vi "Scanner Box Setup.vi"(8 "error in":errorcluster, 11 "VISA resource name":refnum<visa-resource-name>) -> (0 "error out":errorcluster, 3 "VISA resource name out":refnum<visa-resource-name>)   [LabVIEW 2011, in "GPT-9000.lvlib"]
uses:
  <instrlib>/GPT-9000/GPT-9000.lvlib
panel:
  out "Error Message":string
  out "ID Return String":string
  in  "Clear Error(True)":bool=TRUE
  in  "ID Query (True)":bool=TRUE
  in  "Configure RS232 Baud Rate":u32(ring)=115200 items=["9600"=9600, "19200"=19200, "38400"=38400, "57600"=57600, "115200"=115200]
  out "Return the Lo Set Value":u32 format="%08x"
  out "Return the Hi Set Value":u32 format="%08x"
  in  "Number for MANU":i32=1 min=1 max=100 step=1
  in  "CH8_4":enum32{"HI", "LO", "OFF"}(radio)=enum."OFF" caption="CH8"
  in  "CH7_4":enum32{"HI", "LO", "OFF"}(radio)=enum."OFF" caption="CH7"
  in  "CH6_4":enum32{"HI", "LO", "OFF"}(radio)=enum."OFF" caption="CH6"
  in  "CH5_4":enum32{"HI", "LO", "OFF"}(radio)=enum."OFF" caption="CH5"
  in  "CH4_4":enum32{"HI", "LO", "OFF"}(radio)=enum."OFF" caption="CH4"
  in  "CH3_4":enum32{"HI", "LO", "OFF"}(radio)=enum."OFF" caption="CH3"
  in  "CH2_4":enum32{"HI", "LO", "OFF"}(radio)=enum."OFF" caption="CH2"
  in  "CH1_4":enum32{"HI", "LO", "OFF"}(radio)=enum."OFF" caption="CH1"
  in  "CH8_3":enum32{"HI", "LO", "OFF"}(radio)=enum."OFF" caption="CH8"
  in  "CH7_3":enum32{"HI", "LO", "OFF"}(radio)=enum."OFF" caption="CH7"
  in  "CH6_3":enum32{"HI", "LO", "OFF"}(radio)=enum."OFF" caption="CH6"
  in  "CH5_3":enum32{"HI", "LO", "OFF"}(radio)=enum."OFF" caption="CH5"
  in  "CH4_3":enum32{"HI", "LO", "OFF"}(radio)=enum."OFF" caption="CH4"
  in  "CH3_3":enum32{"HI", "LO", "OFF"}(radio)=enum."OFF" caption="CH3"
  in  "CH2_3":enum32{"HI", "LO", "OFF"}(radio)=enum."OFF" caption="CH2"
  in  "CH1_3":enum32{"HI", "LO", "OFF"}(radio)=enum."OFF" caption="CH1"
  in  "CH8_2":enum32{"HI", "LO", "OFF"}(radio)=enum."OFF" caption="CH8"
  in  "CH7_2":enum32{"HI", "LO", "OFF"}(radio)=enum."OFF" caption="CH7"
  in  "CH6_2":enum32{"HI", "LO", "OFF"}(radio)=enum."OFF" caption="CH6"
  in  "CH5_2":enum32{"HI", "LO", "OFF"}(radio)=enum."OFF" caption="CH5"
  in  "CH4_2":enum32{"HI", "LO", "OFF"}(radio)=enum."OFF" caption="CH4"
  in  "CH3_2":enum32{"HI", "LO", "OFF"}(radio)=enum."OFF" caption="CH3"
  in  "CH2_2":enum32{"HI", "LO", "OFF"}(radio)=enum."OFF" caption="CH2"
  in  "CH1_2":enum32{"HI", "LO", "OFF"}(radio)=enum."OFF" caption="CH1"
  in  "CH8_1":enum32{"HI", "LO", "OFF"}(radio)=enum."OFF" caption="CH8"
  in  "CH7_1":enum32{"HI", "LO", "OFF"}(radio)=enum."OFF" caption="CH7"
  in  "CH6_1":enum32{"HI", "LO", "OFF"}(radio)=enum."OFF" caption="CH6"
  in  "CH5_1":enum32{"HI", "LO", "OFF"}(radio)=enum."OFF" caption="CH5"
  in  "CH4_1":enum32{"HI", "LO", "OFF"}(radio)=enum."OFF" caption="CH4"
  in  "CH3_1":enum32{"HI", "LO", "OFF"}(radio)=enum."OFF" caption="CH3"
  in  "CH2_1":enum32{"HI", "LO", "OFF"}(radio)=enum."OFF" caption="CH2"
  in  "CH1_1":enum32{"HI", "LO", "OFF"}(radio)=enum."OFF" caption="CH1"
  # "BOX(1ST)"
  # "BOX(2ND)"
  # "BOX(3RD)"
  # "BOX(4TH)"
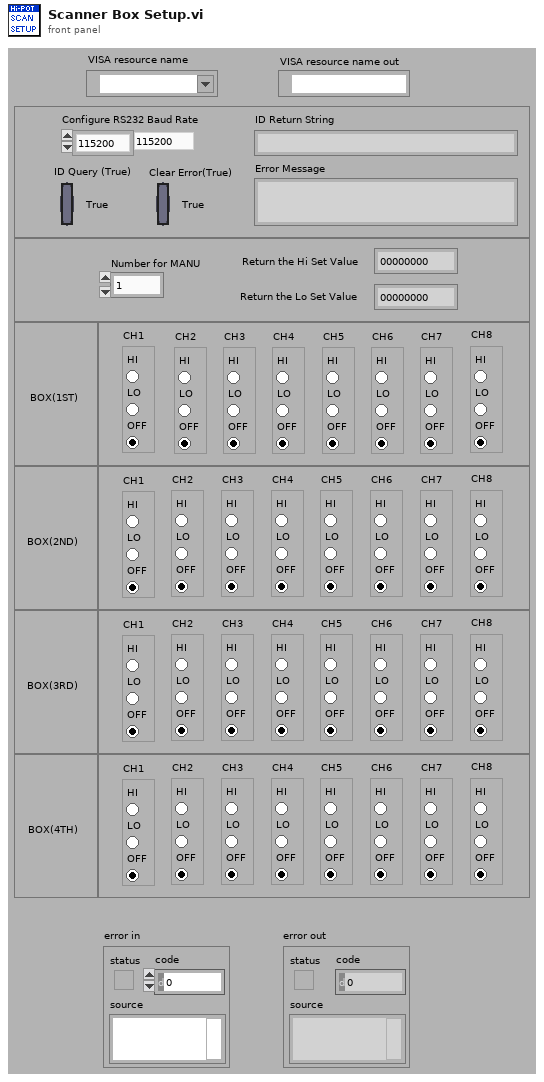
[diagram p1: front panel]
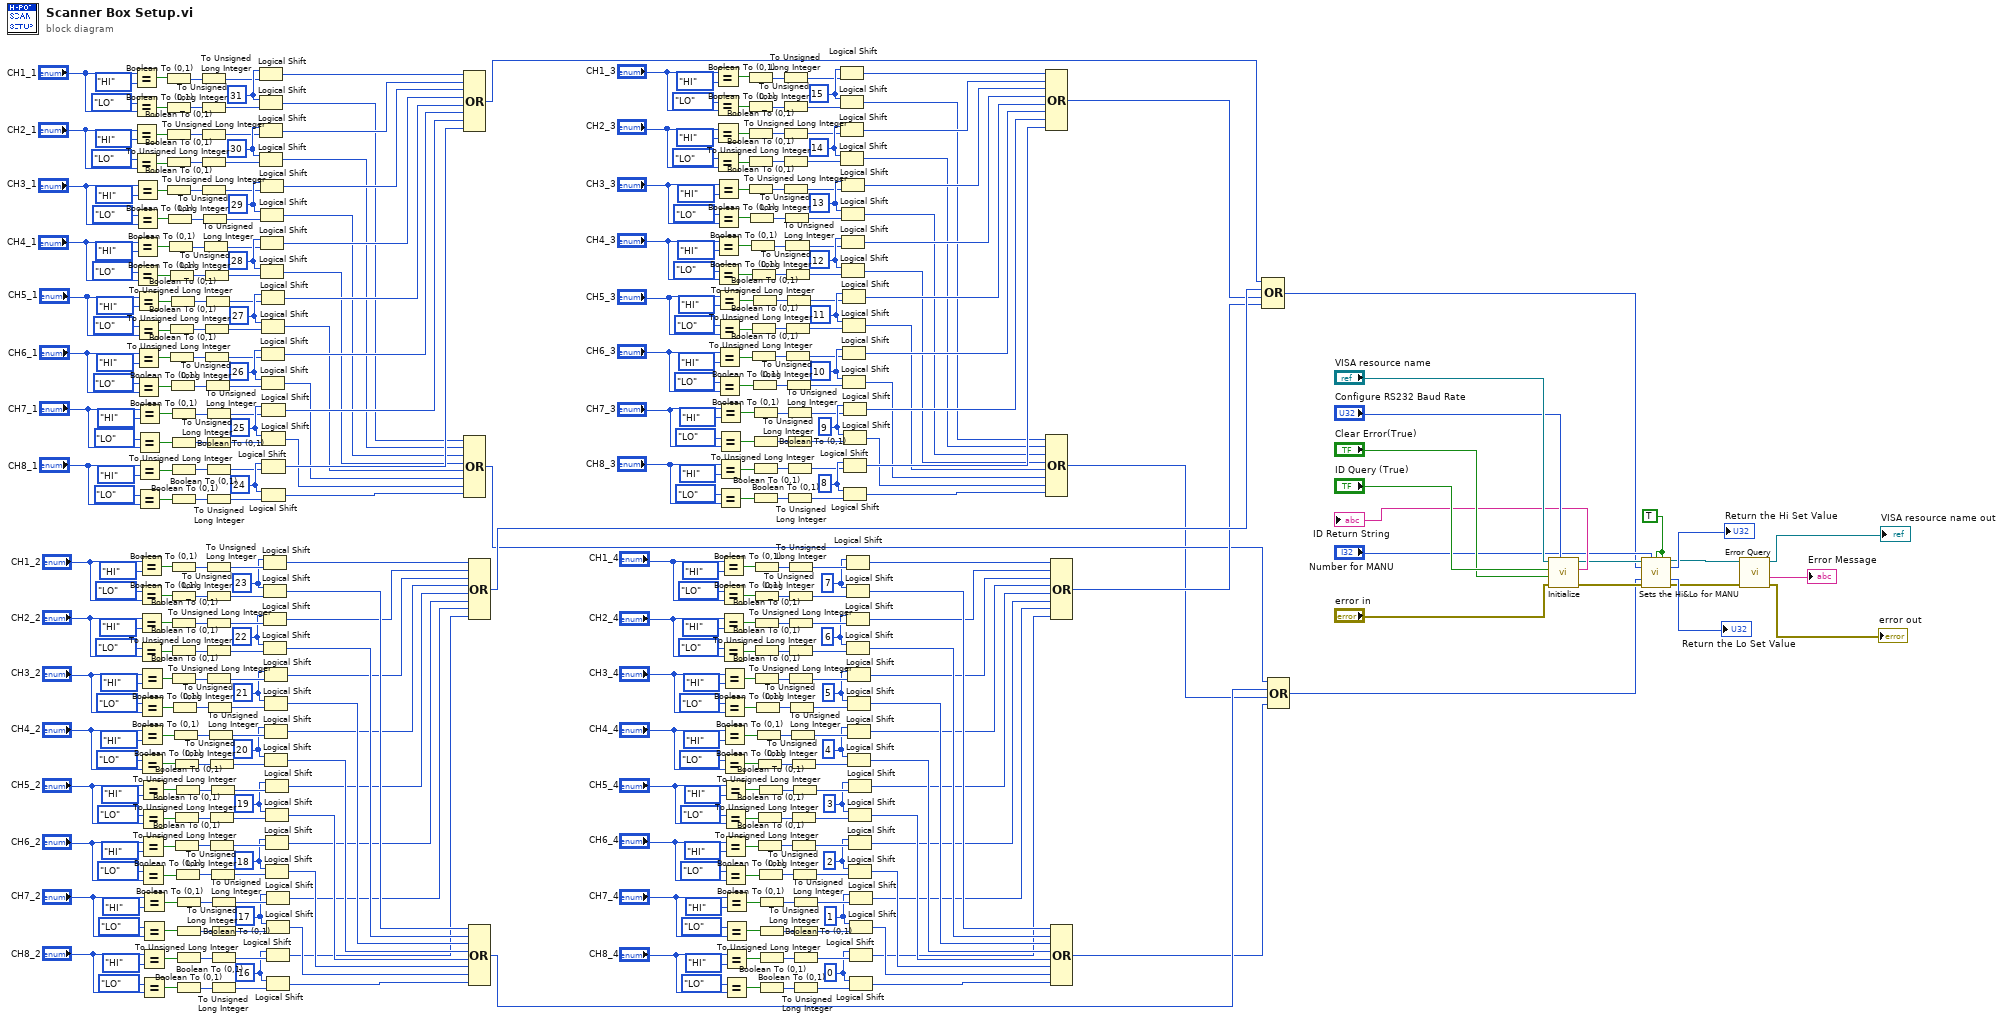
[diagram p0: block diagram]
diagram:
  w8 = TRUE
  w50 = i8 0 ("y")
  w49 = i8 1 ("y")
  w55 = i8 2 ("y")
  w56 = i8 3 ("y")
  w43 = i8 4 ("y")
  w44 = i8 5 ("y")
  w38 = i8 6 ("y")
  w75 = u8 7 ("y")
  w205 = i8 8 ("y")
  w206 = i8 9 ("y")
  w200 = i8 10 ("y")
  w199 = i8 11 ("y")
  w212 = i8 12 ("y")
  w211 = i8 13 ("y")
  w217 = i8 14 ("y")
  w180 = u8 15 ("y")
  w242 = i8 16 ("y")
  w241 = i8 17 ("y")
  w247 = i8 18 ("y")
  w248 = i8 19 ("y")
  w235 = i8 20 ("y")
  w236 = i8 21 ("y")
  w230 = i8 22 ("y")
  w267 = u8 23 ("y")
  w393 = i8 24 ("y")
  w394 = i8 25 ("y")
  w388 = i8 26 ("y")
  w387 = i8 27 ("y")
  w402 = i8 28 ("y")
  w401 = i8 29 ("y")
  w408 = i8 30 ("y")
  w364 = u8 31 ("y")
  n1 = Equal?(x="CH1_1", y=enum32{"HI", "LO", "OFF"}."HI") -> (x = y?=w363:bool)
  n2 = Equal?(x=enum32{"HI", "LO", "OFF"}."LO", y="CH1_1") -> (x = y?=w358:bool)
  n3 = Equal?(x="CH2_1", y=enum32{"HI", "LO", "OFF"}."HI") -> (x = y?=w356:bool)
  n4 = Equal?(x=enum32{"HI", "LO", "OFF"}."LO", y="CH2_1") -> (x = y?=w353:bool)
  n5 = Equal?(x="CH3_1", y=enum32{"HI", "LO", "OFF"}."HI") -> (x = y?=w350:bool)
  n6 = Equal?(x=enum32{"HI", "LO", "OFF"}."LO", y="CH3_1") -> (x = y?=w347:bool)
  n7 = Equal?(x="CH4_1", y=enum32{"HI", "LO", "OFF"}."HI") -> (x = y?=w344:bool)
  n8 = Equal?(x=enum32{"HI", "LO", "OFF"}."LO", y="CH4_1") -> (x = y?=w341:bool)
  n9 = Equal?(x="CH5_1", y=enum32{"HI", "LO", "OFF"}."HI") -> (x = y?=w338:bool)
  n10 = Equal?(x=enum32{"HI", "LO", "OFF"}."LO", y="CH5_1") -> (x = y?=w335:bool)
  n11 = Equal?(x="CH6_1", y=enum32{"HI", "LO", "OFF"}."HI") -> (x = y?=w332:bool)
  n12 = Equal?(x=enum32{"HI", "LO", "OFF"}."LO", y="CH6_1") -> (x = y?=w329:bool)
  n13 = Equal?(x="CH7_1", y=enum32{"HI", "LO", "OFF"}."HI") -> (x = y?=w326:bool)
  n14 = Equal?(x=enum32{"HI", "LO", "OFF"}."LO", y="CH7_1") -> (x = y?=w323:bool)
  n15 = Equal?(x="CH8_1", y=enum32{"HI", "LO", "OFF"}."HI") -> (x = y?=w320:bool)
  n16 = Equal?(x=enum32{"HI", "LO", "OFF"}."LO", y="CH8_1") -> (x = y?=w317:bool)
  n17 = Equal?(x="CH1_2", y=enum32{"HI", "LO", "OFF"}."HI") -> (x = y?=w268:bool)
  n18 = Equal?(x=enum32{"HI", "LO", "OFF"}."LO", y="CH1_2") -> (x = y?=w273:bool)
  n19 = Equal?(x="CH2_2", y=enum32{"HI", "LO", "OFF"}."HI") -> (x = y?=w275:bool)
  n20 = Equal?(x=enum32{"HI", "LO", "OFF"}."LO", y="CH2_2") -> (x = y?=w278:bool)
  n21 = Equal?(x="CH3_2", y=enum32{"HI", "LO", "OFF"}."HI") -> (x = y?=w281:bool)
  n22 = Equal?(x=enum32{"HI", "LO", "OFF"}."LO", y="CH3_2") -> (x = y?=w284:bool)
  n23 = Equal?(x="CH4_2", y=enum32{"HI", "LO", "OFF"}."HI") -> (x = y?=w287:bool)
  n24 = Equal?(x=enum32{"HI", "LO", "OFF"}."LO", y="CH4_2") -> (x = y?=w290:bool)
  n25 = Equal?(x="CH5_2", y=enum32{"HI", "LO", "OFF"}."HI") -> (x = y?=w293:bool)
  n26 = Equal?(x=enum32{"HI", "LO", "OFF"}."LO", y="CH5_2") -> (x = y?=w296:bool)
  n27 = Equal?(x="CH6_2", y=enum32{"HI", "LO", "OFF"}."HI") -> (x = y?=w299:bool)
  n28 = Equal?(x=enum32{"HI", "LO", "OFF"}."LO", y="CH6_2") -> (x = y?=w302:bool)
  n29 = Equal?(x="CH7_2", y=enum32{"HI", "LO", "OFF"}."HI") -> (x = y?=w305:bool)
  n30 = Equal?(x=enum32{"HI", "LO", "OFF"}."LO", y="CH7_2") -> (x = y?=w308:bool)
  n31 = Equal?(x="CH8_2", y=enum32{"HI", "LO", "OFF"}."HI") -> (x = y?=w311:bool)
  n32 = Equal?(x=enum32{"HI", "LO", "OFF"}."LO", y="CH8_2") -> (x = y?=w314:bool)
  n33 = Boolean To (0,1)(Boolean=w363) -> (0, 1=w362:i16)
  n34 = Boolean To (0,1)(Boolean=w358) -> (0, 1=w360:i16)
  n35 = Boolean To (0,1)(Boolean=w356) -> (0, 1=w357:i16)
  n36 = Boolean To (0,1)(Boolean=w353) -> (0, 1=w354:i16)
  n37 = Boolean To (0,1)(Boolean=w350) -> (0, 1=w351:i16)
  n38 = Boolean To (0,1)(Boolean=w347) -> (0, 1=w348:i16)
  n39 = Boolean To (0,1)(Boolean=w344) -> (0, 1=w345:i16)
  n40 = Boolean To (0,1)(Boolean=w341) -> (0, 1=w342:i16)
  n41 = Boolean To (0,1)(Boolean=w335) -> (0, 1=w336:i16)
  n42 = Boolean To (0,1)(Boolean=w332) -> (0, 1=w333:i16)
  n43 = Boolean To (0,1)(Boolean=w338) -> (0, 1=w339:i16)
  n44 = Boolean To (0,1)(Boolean=w329) -> (0, 1=w330:i16)
  n45 = Boolean To (0,1)(Boolean=w326) -> (0, 1=w327:i16)
  n46 = Boolean To (0,1)(Boolean=w323) -> (0, 1=w324:i16)
  n47 = Boolean To (0,1)(Boolean=w320) -> (0, 1=w321:i16)
  n48 = Boolean To (0,1)(Boolean=w317) -> (0, 1=w318:i16)
  n49 = Boolean To (0,1)(Boolean=w268) -> (0, 1=w269:i16)
  n50 = Boolean To (0,1)(Boolean=w273) -> (0, 1=w271:i16)
  n51 = Boolean To (0,1)(Boolean=w275) -> (0, 1=w274:i16)
  n52 = Boolean To (0,1)(Boolean=w278) -> (0, 1=w277:i16)
  n53 = Boolean To (0,1)(Boolean=w281) -> (0, 1=w280:i16)
  n54 = Boolean To (0,1)(Boolean=w284) -> (0, 1=w283:i16)
  n55 = Boolean To (0,1)(Boolean=w287) -> (0, 1=w286:i16)
  n56 = Boolean To (0,1)(Boolean=w290) -> (0, 1=w289:i16)
  n57 = Boolean To (0,1)(Boolean=w296) -> (0, 1=w295:i16)
  n58 = Boolean To (0,1)(Boolean=w299) -> (0, 1=w298:i16)
  n59 = Boolean To (0,1)(Boolean=w293) -> (0, 1=w292:i16)
  n60 = Boolean To (0,1)(Boolean=w302) -> (0, 1=w301:i16)
  n61 = Boolean To (0,1)(Boolean=w305) -> (0, 1=w304:i16)
  n62 = Boolean To (0,1)(Boolean=w308) -> (0, 1=w307:i16)
  n63 = Boolean To (0,1)(Boolean=w311) -> (0, 1=w310:i16)
  n64 = Boolean To (0,1)(Boolean=w314) -> (0, 1=w313:i16)
  n65 = To Unsigned Long Integer(number=w362) -> (unsigned 32bit integer=w361:u32)
  n66 = To Unsigned Long Integer(number=w360) -> (unsigned 32bit integer=w359:u32)
  n67 = To Unsigned Long Integer(number=w357) -> (unsigned 32bit integer=w355:u32)
  n68 = To Unsigned Long Integer(number=w354) -> (unsigned 32bit integer=w352:u32)
  n69 = To Unsigned Long Integer(number=w351) -> (unsigned 32bit integer=w349:u32)
  n70 = To Unsigned Long Integer(number=w348) -> (unsigned 32bit integer=w346:u32)
  n71 = To Unsigned Long Integer(number=w345) -> (unsigned 32bit integer=w343:u32)
  n72 = To Unsigned Long Integer(number=w342) -> (unsigned 32bit integer=w340:u32)
  n73 = To Unsigned Long Integer(number=w336) -> (unsigned 32bit integer=w334:u32)
  n74 = To Unsigned Long Integer(number=w333) -> (unsigned 32bit integer=w331:u32)
  n75 = To Unsigned Long Integer(number=w339) -> (unsigned 32bit integer=w337:u32)
  n76 = To Unsigned Long Integer(number=w330) -> (unsigned 32bit integer=w328:u32)
  n77 = To Unsigned Long Integer(number=w327) -> (unsigned 32bit integer=w325:u32)
  n78 = To Unsigned Long Integer(number=w324) -> (unsigned 32bit integer=w322:u32)
  n79 = To Unsigned Long Integer(number=w321) -> (unsigned 32bit integer=w319:u32)
  n80 = To Unsigned Long Integer(number=w318) -> (unsigned 32bit integer=w316:u32)
  n81 = To Unsigned Long Integer(number=w269) -> (unsigned 32bit integer=w270:u32)
  n82 = To Unsigned Long Integer(number=w271) -> (unsigned 32bit integer=w272:u32)
  n83 = To Unsigned Long Integer(number=w274) -> (unsigned 32bit integer=w276:u32)
  n84 = To Unsigned Long Integer(number=w277) -> (unsigned 32bit integer=w279:u32)
  n85 = To Unsigned Long Integer(number=w280) -> (unsigned 32bit integer=w282:u32)
  n86 = To Unsigned Long Integer(number=w283) -> (unsigned 32bit integer=w285:u32)
  n87 = To Unsigned Long Integer(number=w286) -> (unsigned 32bit integer=w288:u32)
  n88 = To Unsigned Long Integer(number=w289) -> (unsigned 32bit integer=w291:u32)
  n89 = To Unsigned Long Integer(number=w295) -> (unsigned 32bit integer=w297:u32)
  n90 = To Unsigned Long Integer(number=w298) -> (unsigned 32bit integer=w300:u32)
  n91 = To Unsigned Long Integer(number=w292) -> (unsigned 32bit integer=w294:u32)
  n92 = To Unsigned Long Integer(number=w301) -> (unsigned 32bit integer=w303:u32)
  n93 = To Unsigned Long Integer(number=w304) -> (unsigned 32bit integer=w306:u32)
  n94 = To Unsigned Long Integer(number=w307) -> (unsigned 32bit integer=w309:u32)
  n95 = To Unsigned Long Integer(number=w310) -> (unsigned 32bit integer=w312:u32)
  n96 = To Unsigned Long Integer(number=w313) -> (unsigned 32bit integer=w315:u32)
  n97 = Logical Shift(y=w364, x=w361) -> (x << y=w380:u32)
  n98 = Logical Shift(y=w364, x=w359) -> (x << y=w365:u32)
  n99 = Logical Shift(y=w408, x=w355) -> (x << y=w379:u32)
  n100 = Logical Shift(y=w408, x=w352) -> (x << y=w366:u32)
  n101 = Logical Shift(y=w401, x=w349) -> (x << y=w378:u32)
  n102 = Logical Shift(y=w401, x=w346) -> (x << y=w367:u32)
  n103 = Logical Shift(y=w402, x=w343) -> (x << y=w377:u32)
  n104 = Logical Shift(y=w402, x=w340) -> (x << y=w368:u32)
  n105 = Logical Shift(y=w387, x=w337) -> (x << y=w376:u32)
  n106 = Logical Shift(y=w387, x=w334) -> (x << y=w369:u32)
  n107 = Logical Shift(y=w388, x=w331) -> (x << y=w375:u32)
  n108 = Logical Shift(y=w388, x=w328) -> (x << y=w370:u32)
  n109 = Logical Shift(y=w394, x=w325) -> (x << y=w374:u32)
  n110 = Logical Shift(y=w394, x=w322) -> (x << y=w371:u32)
  n111 = Logical Shift(y=w393, x=w319) -> (x << y=w373:u32)
  n112 = Logical Shift(y=w393, x=w316) -> (x << y=w372:u32)
  n113 = Logical Shift(y=w267, x=w270) -> (x << y=w251:u32)
  n114 = Logical Shift(y=w267, x=w272) -> (x << y=w266:u32)
  n115 = Logical Shift(y=w230, x=w276) -> (x << y=w252:u32)
  n116 = Logical Shift(y=w230, x=w279) -> (x << y=w265:u32)
  n117 = Logical Shift(y=w236, x=w282) -> (x << y=w253:u32)
  n118 = Logical Shift(y=w236, x=w285) -> (x << y=w264:u32)
  n119 = Logical Shift(y=w235, x=w288) -> (x << y=w254:u32)
  n120 = Logical Shift(y=w235, x=w291) -> (x << y=w263:u32)
  n121 = Logical Shift(y=w248, x=w294) -> (x << y=w255:u32)
  n122 = Logical Shift(y=w248, x=w297) -> (x << y=w262:u32)
  n123 = Logical Shift(y=w247, x=w300) -> (x << y=w256:u32)
  n124 = Logical Shift(y=w247, x=w303) -> (x << y=w261:u32)
  n125 = Logical Shift(y=w241, x=w306) -> (x << y=w257:u32)
  n126 = Logical Shift(y=w241, x=w309) -> (x << y=w260:u32)
  n127 = Logical Shift(y=w242, x=w312) -> (x << y=w258:u32)
  n128 = Logical Shift(y=w242, x=w315) -> (x << y=w259:u32)
  n129 = Compound Arithmetic op=OR(w380, w379, w378, w377, w376, w375, w374, w373) -> (w27:u32)
  n130 = Compound Arithmetic op=OR(w365, w366, w367, w368, w369, w370, w371, w372) -> (w23:u32)
  n131 = Compound Arithmetic op=OR(w251, w252, w253, w254, w255, w256, w257, w258) -> (w26:u32)
  n132 = Compound Arithmetic op=OR(w266, w265, w264, w263, w262, w261, w260, w259) -> (w22:u32)
  n133 = Equal?(x="CH1_3", y=enum32{"HI", "LO", "OFF"}."HI") -> (x = y?=w179:bool)
  n134 = Equal?(x=enum32{"HI", "LO", "OFF"}."LO", y="CH1_3") -> (x = y?=w174:bool)
  n135 = Equal?(x="CH2_3", y=enum32{"HI", "LO", "OFF"}."HI") -> (x = y?=w172:bool)
  n136 = Equal?(x=enum32{"HI", "LO", "OFF"}."LO", y="CH2_3") -> (x = y?=w169:bool)
  n137 = Equal?(x="CH3_3", y=enum32{"HI", "LO", "OFF"}."HI") -> (x = y?=w166:bool)
  n138 = Equal?(x=enum32{"HI", "LO", "OFF"}."LO", y="CH3_3") -> (x = y?=w163:bool)
  n139 = Equal?(x="CH4_3", y=enum32{"HI", "LO", "OFF"}."HI") -> (x = y?=w160:bool)
  n140 = Equal?(x=enum32{"HI", "LO", "OFF"}."LO", y="CH4_3") -> (x = y?=w157:bool)
  n141 = Equal?(x="CH5_3", y=enum32{"HI", "LO", "OFF"}."HI") -> (x = y?=w154:bool)
  n142 = Equal?(x=enum32{"HI", "LO", "OFF"}."LO", y="CH5_3") -> (x = y?=w151:bool)
  n143 = Equal?(x="CH6_3", y=enum32{"HI", "LO", "OFF"}."HI") -> (x = y?=w148:bool)
  n144 = Equal?(x=enum32{"HI", "LO", "OFF"}."LO", y="CH6_3") -> (x = y?=w145:bool)
  n145 = Equal?(x="CH7_3", y=enum32{"HI", "LO", "OFF"}."HI") -> (x = y?=w142:bool)
  n146 = Equal?(x=enum32{"HI", "LO", "OFF"}."LO", y="CH7_3") -> (x = y?=w139:bool)
  n147 = Equal?(x="CH8_3", y=enum32{"HI", "LO", "OFF"}."HI") -> (x = y?=w136:bool)
  n148 = Equal?(x=enum32{"HI", "LO", "OFF"}."LO", y="CH8_3") -> (x = y?=w133:bool)
  n149 = Equal?(x="CH1_4", y=enum32{"HI", "LO", "OFF"}."HI") -> (x = y?=w76:bool)
  n150 = Equal?(x=enum32{"HI", "LO", "OFF"}."LO", y="CH1_4") -> (x = y?=w81:bool)
  n151 = Equal?(x="CH2_4", y=enum32{"HI", "LO", "OFF"}."HI") -> (x = y?=w83:bool)
  n152 = Equal?(x=enum32{"HI", "LO", "OFF"}."LO", y="CH2_4") -> (x = y?=w86:bool)
  n153 = Equal?(x="CH3_4", y=enum32{"HI", "LO", "OFF"}."HI") -> (x = y?=w89:bool)
  n154 = Equal?(x=enum32{"HI", "LO", "OFF"}."LO", y="CH3_4") -> (x = y?=w92:bool)
  n155 = Equal?(x="CH4_4", y=enum32{"HI", "LO", "OFF"}."HI") -> (x = y?=w95:bool)
  n156 = Equal?(x=enum32{"HI", "LO", "OFF"}."LO", y="CH4_4") -> (x = y?=w98:bool)
  n157 = Equal?(x="CH5_4", y=enum32{"HI", "LO", "OFF"}."HI") -> (x = y?=w101:bool)
  n158 = Equal?(x=enum32{"HI", "LO", "OFF"}."LO", y="CH5_4") -> (x = y?=w104:bool)
  n159 = Equal?(x="CH6_4", y=enum32{"HI", "LO", "OFF"}."HI") -> (x = y?=w107:bool)
  n160 = Equal?(x=enum32{"HI", "LO", "OFF"}."LO", y="CH6_4") -> (x = y?=w110:bool)
  n161 = Equal?(x="CH7_4", y=enum32{"HI", "LO", "OFF"}."HI") -> (x = y?=w113:bool)
  n162 = Equal?(x=enum32{"HI", "LO", "OFF"}."LO", y="CH7_4") -> (x = y?=w116:bool)
  n163 = Equal?(x="CH8_4", y=enum32{"HI", "LO", "OFF"}."HI") -> (x = y?=w119:bool)
  n164 = Equal?(x=enum32{"HI", "LO", "OFF"}."LO", y="CH8_4") -> (x = y?=w122:bool)
  n165 = Boolean To (0,1)(Boolean=w179) -> (0, 1=w178:i16)
  n166 = Boolean To (0,1)(Boolean=w174) -> (0, 1=w176:i16)
  n167 = Boolean To (0,1)(Boolean=w172) -> (0, 1=w173:i16)
  n168 = Boolean To (0,1)(Boolean=w169) -> (0, 1=w170:i16)
  n169 = Boolean To (0,1)(Boolean=w166) -> (0, 1=w167:i16)
  n170 = Boolean To (0,1)(Boolean=w163) -> (0, 1=w164:i16)
  n171 = Boolean To (0,1)(Boolean=w160) -> (0, 1=w161:i16)
  n172 = Boolean To (0,1)(Boolean=w157) -> (0, 1=w158:i16)
  n173 = Boolean To (0,1)(Boolean=w151) -> (0, 1=w152:i16)
  n174 = Boolean To (0,1)(Boolean=w148) -> (0, 1=w149:i16)
  n175 = Boolean To (0,1)(Boolean=w154) -> (0, 1=w155:i16)
  n176 = Boolean To (0,1)(Boolean=w145) -> (0, 1=w146:i16)
  n177 = Boolean To (0,1)(Boolean=w142) -> (0, 1=w143:i16)
  n178 = Boolean To (0,1)(Boolean=w139) -> (0, 1=w140:i16)
  n179 = Boolean To (0,1)(Boolean=w136) -> (0, 1=w137:i16)
  n180 = Boolean To (0,1)(Boolean=w133) -> (0, 1=w134:i16)
  n181 = Boolean To (0,1)(Boolean=w76) -> (0, 1=w77:i16)
  n182 = Boolean To (0,1)(Boolean=w81) -> (0, 1=w79:i16)
  n183 = Boolean To (0,1)(Boolean=w83) -> (0, 1=w82:i16)
  n184 = Boolean To (0,1)(Boolean=w86) -> (0, 1=w85:i16)
  n185 = Boolean To (0,1)(Boolean=w89) -> (0, 1=w88:i16)
  n186 = Boolean To (0,1)(Boolean=w92) -> (0, 1=w91:i16)
  n187 = Boolean To (0,1)(Boolean=w95) -> (0, 1=w94:i16)
  n188 = Boolean To (0,1)(Boolean=w98) -> (0, 1=w97:i16)
  n189 = Boolean To (0,1)(Boolean=w104) -> (0, 1=w103:i16)
  n190 = Boolean To (0,1)(Boolean=w107) -> (0, 1=w106:i16)
  n191 = Boolean To (0,1)(Boolean=w101) -> (0, 1=w100:i16)
  n192 = Boolean To (0,1)(Boolean=w110) -> (0, 1=w109:i16)
  n193 = Boolean To (0,1)(Boolean=w113) -> (0, 1=w112:i16)
  n194 = Boolean To (0,1)(Boolean=w116) -> (0, 1=w115:i16)
  n195 = Boolean To (0,1)(Boolean=w119) -> (0, 1=w118:i16)
  n196 = Boolean To (0,1)(Boolean=w122) -> (0, 1=w121:i16)
  n197 = To Unsigned Long Integer(number=w178) -> (unsigned 32bit integer=w177:u32)
  n198 = To Unsigned Long Integer(number=w176) -> (unsigned 32bit integer=w175:u32)
  n199 = To Unsigned Long Integer(number=w173) -> (unsigned 32bit integer=w171:u32)
  n200 = To Unsigned Long Integer(number=w170) -> (unsigned 32bit integer=w168:u32)
  n201 = To Unsigned Long Integer(number=w167) -> (unsigned 32bit integer=w165:u32)
  n202 = To Unsigned Long Integer(number=w164) -> (unsigned 32bit integer=w162:u32)
  n203 = To Unsigned Long Integer(number=w161) -> (unsigned 32bit integer=w159:u32)
  n204 = To Unsigned Long Integer(number=w158) -> (unsigned 32bit integer=w156:u32)
  n205 = To Unsigned Long Integer(number=w152) -> (unsigned 32bit integer=w150:u32)
  n206 = To Unsigned Long Integer(number=w149) -> (unsigned 32bit integer=w147:u32)
  n207 = To Unsigned Long Integer(number=w155) -> (unsigned 32bit integer=w153:u32)
  n208 = To Unsigned Long Integer(number=w146) -> (unsigned 32bit integer=w144:u32)
  n209 = To Unsigned Long Integer(number=w143) -> (unsigned 32bit integer=w141:u32)
  n210 = To Unsigned Long Integer(number=w140) -> (unsigned 32bit integer=w138:u32)
  n211 = To Unsigned Long Integer(number=w137) -> (unsigned 32bit integer=w135:u32)
  n212 = To Unsigned Long Integer(number=w134) -> (unsigned 32bit integer=w132:u32)
  n213 = To Unsigned Long Integer(number=w77) -> (unsigned 32bit integer=w78:u32)
  n214 = To Unsigned Long Integer(number=w79) -> (unsigned 32bit integer=w80:u32)
  n215 = To Unsigned Long Integer(number=w82) -> (unsigned 32bit integer=w84:u32)
  n216 = To Unsigned Long Integer(number=w85) -> (unsigned 32bit integer=w87:u32)
  n217 = To Unsigned Long Integer(number=w88) -> (unsigned 32bit integer=w90:u32)
  n218 = To Unsigned Long Integer(number=w91) -> (unsigned 32bit integer=w93:u32)
  n219 = To Unsigned Long Integer(number=w94) -> (unsigned 32bit integer=w96:u32)
  n220 = To Unsigned Long Integer(number=w97) -> (unsigned 32bit integer=w99:u32)
  n221 = To Unsigned Long Integer(number=w103) -> (unsigned 32bit integer=w105:u32)
  n222 = To Unsigned Long Integer(number=w106) -> (unsigned 32bit integer=w108:u32)
  n223 = To Unsigned Long Integer(number=w100) -> (unsigned 32bit integer=w102:u32)
  n224 = To Unsigned Long Integer(number=w109) -> (unsigned 32bit integer=w111:u32)
  n225 = To Unsigned Long Integer(number=w112) -> (unsigned 32bit integer=w114:u32)
  n226 = To Unsigned Long Integer(number=w115) -> (unsigned 32bit integer=w117:u32)
  n227 = To Unsigned Long Integer(number=w118) -> (unsigned 32bit integer=w120:u32)
  n228 = To Unsigned Long Integer(number=w121) -> (unsigned 32bit integer=w123:u32)
  n229 = Logical Shift(y=w180, x=w177) -> (x << y=w196:u32)
  n230 = Logical Shift(y=w180, x=w175) -> (x << y=w181:u32)
  n231 = Logical Shift(y=w217, x=w171) -> (x << y=w195:u32)
  n232 = Logical Shift(y=w217, x=w168) -> (x << y=w182:u32)
  n233 = Logical Shift(y=w211, x=w165) -> (x << y=w194:u32)
  n234 = Logical Shift(y=w211, x=w162) -> (x << y=w183:u32)
  n235 = Logical Shift(y=w212, x=w159) -> (x << y=w193:u32)
  n236 = Logical Shift(y=w212, x=w156) -> (x << y=w184:u32)
  n237 = Logical Shift(y=w199, x=w153) -> (x << y=w192:u32)
  n238 = Logical Shift(y=w199, x=w150) -> (x << y=w185:u32)
  n239 = Logical Shift(y=w200, x=w147) -> (x << y=w191:u32)
  n240 = Logical Shift(y=w200, x=w144) -> (x << y=w186:u32)
  n241 = Logical Shift(y=w206, x=w141) -> (x << y=w190:u32)
  n242 = Logical Shift(y=w206, x=w138) -> (x << y=w187:u32)
  n243 = Logical Shift(y=w205, x=w135) -> (x << y=w189:u32)
  n244 = Logical Shift(y=w205, x=w132) -> (x << y=w188:u32)
  n245 = Logical Shift(y=w75, x=w78) -> (x << y=w59:u32)
  n246 = Logical Shift(y=w75, x=w80) -> (x << y=w74:u32)
  n247 = Logical Shift(y=w38, x=w84) -> (x << y=w60:u32)
  n248 = Logical Shift(y=w38, x=w87) -> (x << y=w73:u32)
  n249 = Logical Shift(y=w44, x=w90) -> (x << y=w61:u32)
  n250 = Logical Shift(y=w44, x=w93) -> (x << y=w72:u32)
  n251 = Logical Shift(y=w43, x=w96) -> (x << y=w62:u32)
  n252 = Logical Shift(y=w43, x=w99) -> (x << y=w71:u32)
  n253 = Logical Shift(y=w56, x=w102) -> (x << y=w63:u32)
  n254 = Logical Shift(y=w56, x=w105) -> (x << y=w70:u32)
  n255 = Logical Shift(y=w55, x=w108) -> (x << y=w64:u32)
  n256 = Logical Shift(y=w55, x=w111) -> (x << y=w69:u32)
  n257 = Logical Shift(y=w49, x=w114) -> (x << y=w65:u32)
  n258 = Logical Shift(y=w49, x=w117) -> (x << y=w68:u32)
  n259 = Logical Shift(y=w50, x=w120) -> (x << y=w66:u32)
  n260 = Logical Shift(y=w50, x=w123) -> (x << y=w67:u32)
  n261 = Compound Arithmetic op=OR(w196, w195, w194, w193, w192, w191, w190, w189) -> (w25:u32)
  n262 = Compound Arithmetic op=OR(w181, w182, w183, w184, w185, w186, w187, w188) -> (w21:u32)
  n263 = Compound Arithmetic op=OR(w59, w60, w61, w62, w63, w64, w65, w66) -> (w24:u32)
  n264 = Compound Arithmetic op=OR(w74, w73, w72, w71, w70, w69, w68, w67) -> (w20:u32)
  n265 = Compound Arithmetic op=OR(w27, w26, w25, w24) -> (w10:u32)
  n266 = Compound Arithmetic op=OR(w23, w22, w21, w20) -> (w9:u32)
  n267 = call <instrlib>:"Initialize.vi"("Configure RS232 Baud Rate"="Configure RS232 Baud Rate", "error in (no error)"="error in", "Clear Error(True)"="Clear Error(True)", "ID Query (True)"="ID Query (True)", "VISA resource name"="VISA resource name") -> ("error out"=w12:errorcluster, "ID Return String"=→"ID Return String":string, "VISA resource name out"=w13:refnum<visa-resource-name>)  [unwired: 3 in, 1 out]
  n268 = call <instrlib>:"Sets the Hi&Lo for MANU.vi"("VISA resource name"=w13, "Number of MANU"="Number for MANU", "Enable to Setup"=w8, "Enable to Query"=w8, "Hi Set Value"=w10, "Lo Set Value"=w9, "error in"=w12) -> ("VISA resource name out"=w5:refnum<visa-resource-name>, "Return the Hi Value"=→"Return the Hi Set Value":u32, "Return the Lo Value"=→"Return the Lo Set Value":u32, "error out"=w4:errorcluster)  [unwired: 5 in]
  n269 = call <instrlib>:"Error Query.vi"("error in (no error)"=w4, "VISA resource name"=w5) -> ("error out"=→"error out":errorcluster, "Error Message"=→"Error Message":string, "VISA resource name out"=→"VISA resource name out":refnum<visa-resource-name>)  [unwired: 6 in, 1 out]
